vi "my글로벌.vi"() -> ()   [LabVIEW 2014]
panel:
  in  "Stop":bool
  in  "Data":dbl
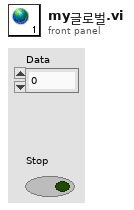
[diagram p1: front panel]
diagram:
